vi "Reorder Array2__ogtk.vi"   [LabVIEW 2020]
doc: "This polymorphic VI reorders 1D and 2D arrays of any size based on the indices you specify. For 2D arrays, it reorders by row or by column."
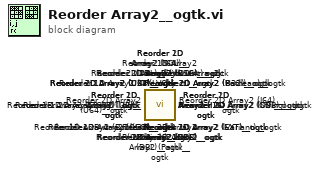
[diagram p0: block diagram]
diagram:
  n1 = call <userlib>:"Reorder 2D Array2 (LVObject)__ogtk.vi"() -> ()  [unwired: 11 in, 1 out]
  n2 = call <userlib>:"Reorder 1D Array2 (LVObject)__ogtk.vi"() -> ()  [unwired: 11 in, 1 out]
  n3 = call <userlib>:"Reorder 2D Array2 (U64)__ogtk.vi"() -> ()  [unwired: 11 in, 1 out]
  n4 = call <userlib>:"Reorder 2D Array2 (I64)__ogtk.vi"() -> ()  [unwired: 11 in, 1 out]
  n5 = call <userlib>:"Reorder 1D Array2 (U64)__ogtk.vi"() -> ()  [unwired: 11 in, 1 out]
  n6 = call <userlib>:"Reorder 1D Array2 (I64)__ogtk.vi"() -> ()  [unwired: 11 in, 1 out]
  n7 = call <userlib>:"Reorder 1D Array2 (Variant)__ogtk.vi"() -> ()  [unwired: 11 in, 1 out]
  n8 = call <userlib>:"Reorder 1D Array2 (Path)__ogtk.vi"() -> ()  [unwired: 11 in, 1 out]
  n9 = call <userlib>:"Reorder 1D Array2 (String)__ogtk.vi"() -> ()  [unwired: 11 in, 1 out]
  n10 = call <userlib>:"Reorder 1D Array2 (Boolean)__ogtk.vi"() -> ()  [unwired: 11 in, 1 out]
  n11 = call <userlib>:"Reorder 1D Array2 (U8)__ogtk.vi"() -> ()  [unwired: 11 in, 1 out]
  n12 = call <userlib>:"Reorder 1D Array2 (U32)__ogtk.vi"() -> ()  [unwired: 11 in, 1 out]
  n13 = call <userlib>:"Reorder 1D Array2 (U16)__ogtk.vi"() -> ()  [unwired: 11 in, 1 out]
  n14 = call <userlib>:"Reorder 1D Array2 (SGL)__ogtk.vi"() -> ()  [unwired: 11 in, 1 out]
  n15 = call <userlib>:"Reorder 1D Array2 (I8)__ogtk.vi"() -> ()  [unwired: 11 in, 1 out]
  n16 = call <userlib>:"Reorder 1D Array2 (I32)__ogtk.vi"() -> ()  [unwired: 11 in, 1 out]
  n17 = call <userlib>:"Reorder 1D Array2 (I16)__ogtk.vi"() -> ()  [unwired: 11 in, 1 out]
  n18 = call <userlib>:"Reorder 1D Array2 (EXT)__ogtk.vi"() -> ()  [unwired: 11 in, 1 out]
  n19 = call <userlib>:"Reorder 1D Array2 (DBL)__ogtk.vi"() -> ()  [unwired: 11 in, 1 out]
  n20 = call <userlib>:"Reorder 1D Array2 (CSG)__ogtk.vi"() -> ()  [unwired: 11 in, 1 out]
  n21 = call <userlib>:"Reorder 1D Array2 (CXT)__ogtk.vi"() -> ()  [unwired: 11 in, 1 out]
  n22 = call <userlib>:"Reorder 1D Array2 (CDB)__ogtk.vi"() -> ()  [unwired: 11 in, 1 out]
  n23 = call <userlib>:"Reorder 2D Array2 (Boolean)__ogtk.vi"() -> ()  [unwired: 11 in, 1 out]
  n24 = call <userlib>:"Reorder 2D Array2 (CDB)__ogtk.vi"() -> ()  [unwired: 11 in, 1 out]
  n25 = call <userlib>:"Reorder 2D Array2 (CSG)__ogtk.vi"() -> ()  [unwired: 11 in, 1 out]
  n26 = call <userlib>:"Reorder 2D Array2 (CXT)__ogtk.vi"() -> ()  [unwired: 11 in, 1 out]
  n27 = call <userlib>:"Reorder 2D Array2 (DBL)__ogtk.vi"() -> ()  [unwired: 11 in, 1 out]
  n28 = call <userlib>:"Reorder 2D Array2 (EXT)__ogtk.vi"() -> ()  [unwired: 11 in, 1 out]
  n29 = call <userlib>:"Reorder 2D Array2 (I8)__ogtk.vi"() -> ()  [unwired: 11 in, 1 out]
  n30 = call <userlib>:"Reorder 2D Array2 (I16)__ogtk.vi"() -> ()  [unwired: 11 in, 1 out]
  n31 = call <userlib>:"Reorder 2D Array2 (I32)__ogtk.vi"() -> ()  [unwired: 11 in, 1 out]
  n32 = call <userlib>:"Reorder 2D Array2 (Path)__ogtk.vi"() -> ()  [unwired: 11 in, 1 out]
  n33 = call <userlib>:"Reorder 2D Array2 (SGL)__ogtk.vi"() -> ()  [unwired: 11 in, 1 out]
  n34 = call <userlib>:"Reorder 2D Array2 (String)__ogtk.vi"() -> ()  [unwired: 11 in, 1 out]
  n35 = call <userlib>:"Reorder 2D Array2 (U8)__ogtk.vi"() -> ()  [unwired: 11 in, 1 out]
  n36 = call <userlib>:"Reorder 2D Array2 (U16)__ogtk.vi"() -> ()  [unwired: 11 in, 1 out]
  n37 = call <userlib>:"Reorder 2D Array2 (U32)__ogtk.vi"() -> ()  [unwired: 11 in, 1 out]
  n38 = call <userlib>:"Reorder 2D Array2 (Variant)__ogtk.vi"() -> ()  [unwired: 11 in, 1 out]
